vi "Teleop.vi"(10 "Match Info":T1={"Autonomous Elapsed Seconds"=0.0, "TeleOp Elapsed Seconds"=0.0, "Disabled Elapsed Seconds"=0.0, "Visited Autonomous"=FALSE, "Visited TeleOp"=FALSE, "Visited Disabled"=FALSE, "Autonomous Settings"={"Autonomous Style"=enum."Independent", "VI Refnum"=refnum}}, 11 "Call Context":T2) -> ()   [LabVIEW 2016]
doc: "This VI is called for each TeleOp packet received from the DS where the robot is not disabled. It is often used to read from the joysticks and update I/O or to update setpoints for timed control loops. It should complete and return within 20 milliseconds or it may miss DS packets."
uses:
  <vilib>/Rock Robotics/WPI/DriverStation/WPI_DriverStationDerivedRobotMode.ctl
  <vilib>/Rock Robotics/WPI/DriverStation/WPI_DriverStationMatch Info.ctl
  <vilib>/Rock Robotics/WPI/Solenoid/WPI_SolenoidValue.ctl
  <vilib>/Rock Robotics/WPI/Utilities/WPI_GetSetVariantRefNum.vi
  <vilib>/Rock Robotics/Network Tables/NT Read Boolean.vi
  <vilib>/Rock Robotics/WPI/Joystick/WPI_JoystickArcadeMapping.vi
  <vilib>/Rock Robotics/Network Tables/NT Write Number.vi
panel:
  out "Brake is Enabled 6":bool
  out "Brake is Enabled 5":bool
  out "Brake is Enabled 4":bool
  out "Brake is Enabled 3":bool
  out "Brake is Enabled 2":bool
  out "Brake is Enabled":bool
  out "Shift Status":dbl
  # "DRIVER CONTROLS"
  # "This is the number that is multiplied with the joystick output to determine high \ngear turning speed, the lower the number the slower it will turn in high gear."
  # "These numbers controls overall how sensitive the joystick is to turning and foreward\nmovement, the lower the number is the faster it will respond to joystick motion. \nIf the number is 1 then it will move in a linear relationship with the joystick."
  # "This controls the maximum foreward and backwards speed of the robot, if at 1 then\nthe robot can move at max power, if at 0 then the robot cannot move at all."
  # "This turns the ability to use autoshift on/off, if activated it does NOT mean that \nautoshift is always on, it simply means that it can be turned on with buttons 6/11."
  # "This turns the ability to use high gear on/off, if activated it does NOT mean that \nhigh gear is always on, it simply means that it can be turned on with button 1."
  # "This turns on the ability to reverse the direction of the robot with the buttons 8/9."
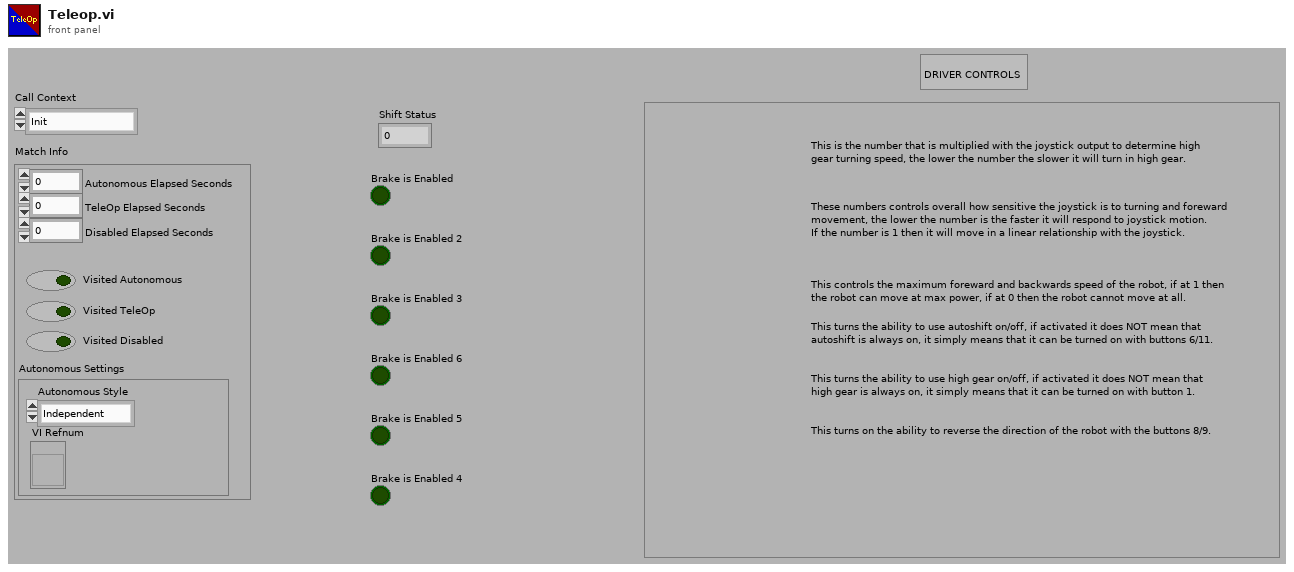
[diagram p1: front panel]
types:
  T1 = typedef "WPI_DriverStationMatch Info.ctl" = cluster{"Autonomous Elapsed Seconds":dbl, "TeleOp Elapsed Seconds":dbl, "Disabled Elapsed Seconds":dbl, "Visited Autonomous":bool, "Visited TeleOp":bool, "Visited Disabled":bool, "Autonomous Settings":cluster{"Autonomous Style":enum16{"Iterative", "Independent"}, "VI Refnum":refnum<vi>}}
  T2 = typedef "WPI_DriverStationDerivedRobotMode.ctl" = enum16{"Init", "Execute", "Stop"}
  T3 = typedef "WPI_JoystickDevRef.ctl" = cluster{"Device":T4}
  T4 = typedef "WPI_JoystickDeviceEnum.ctl" = enum16{"USB 0", "USB 1", "USB 2", "USB 3", "USB 4", "USB 5"}
  T5 = typedef "WPI_MotorControlDeviceRef.ctl" = cluster{"DeviceStatus":errorcluster, "Type":T6, "PWM":cluster{"PWM Channel":T7, "DeadBand":T8}, "CAN":cluster{"Device Number":u8, "SetOutput VI Ref":variant, "GetOutput VI Ref":variant, "Enable VI Ref":variant, "Disable VI Ref":variant, "Data":variant}, "Invert":bool}
  T6 = typedef "WPI_MotorControlType.ctl" = enum16{"PWM", "CAN"}
  T7 = typedef "FPGA_DIOPWMChannel.ctl" = enum8{"PWM 0", "PWM 1", "PWM 2", "PWM 3", "PWM 4", "PWM 5", "PWM 6", "PWM 7", "PWM 8", "PWM 9", "PWM MXP 0", "PWM MXP 1", "PWM MXP 2", "PWM MXP 3", "PWM MXP 4", "PWM MXP 5", "PWM MXP 6", "PWM MXP 7", "PWM MXP 8", "PWM MXP 9", "Invalid"}
  T8 = typedef "WPI_PWMDeadband.ctl" = cluster{"Name":string, "maxPositivePwm":i32, "minPositivePwm":i32, "centerPwm":i32, "maxNegativePwm":i32, "minNegativePwm":i32, "angularRange":u16}
  T9 = typedef "WPI_SolenoidDevRef.ctl" = cluster{"DevStatus":errorcluster, "Pneumatics Control Module":u8, "Forward Solenoid Channel":T10, "Reverse Solenoid Channel":T10}
  T10 = typedef "WPI_SolenoidChannel.ctl" = enum8{"Solenoid 0", "Solenoid 1", "Solenoid 2", "Solenoid 3", "Solenoid 4", "Solenoid 5", "Solenoid 6", "Solenoid 7", "Invalid"}
  T11 = typedef "WPI_CANTalonSRX_GlobalStatus.ctl" = cluster{"Applied Throttle":dbl, "Module Enabled":bool, "CAN Error":errorcluster, "Closed Loop Error":dbl, "Forward Limit Switch Closed":bool, "Reverse Limit Switch Closed":bool, "Sensor Position":dbl, "Sensor Velocity":dbl, "Current":dbl, "Sticky Fault - Over Temp":bool, "Sticky Fault - Under Voltage":bool, "Sticky Fault - Forward Limit":bool, "Sticky Fault - Reverse Limit":bool, "Sticky Fault - Forward Soft Limit":bool, "Sticky Fault - Reverse Soft Limit":bool, "Brake is Enabled":bool, "Encoder Position":dbl, "Encoder Velocity":dbl, "Encoder Index Count":dbl, "Encoder A Pin State":bool, "Encoder B Pin State":bool, "Encoder Index Pin State":bool, "Analog In":dbl, "Analog In Velocity":dbl, "Temperature (C)":dbl, "Battery Voltage":dbl, "Control 5 Is Supported":bool, "Current Profile Slot Select":dbl, "Pos Div 8":bool, "Vel Div 4":bool, "Pulse Width Position":i32, "Pulse Width Velocity":i32, "Pulse Width Rise To Rise (us)":i32, "Pulse Width Rise To Fall (us)":i32, "Mot Prof Active Is Under Run":bool, "Mot Prof Active Has Under Run":bool, "Mot Prof Active Is Last":bool, "Mot Prof Active Velocity Only":bool, "Mot Prof Active Is Valid":bool, "Mot Prof Buffer Is Full":bool, "Mot Prof Active Profile Slot Select":i32, "Mot Prof NextID":i32, "Mot Prof Count":i32, "Mot Prof Active Velocity":dbl, "Mot Prof Active Position":dbl, "Mot Prof Output Enable":i32}
  T12 = typedef "WPI_SolenoidValue.ctl" = enum16{"Off", "On", "Forward", "Reverse"}
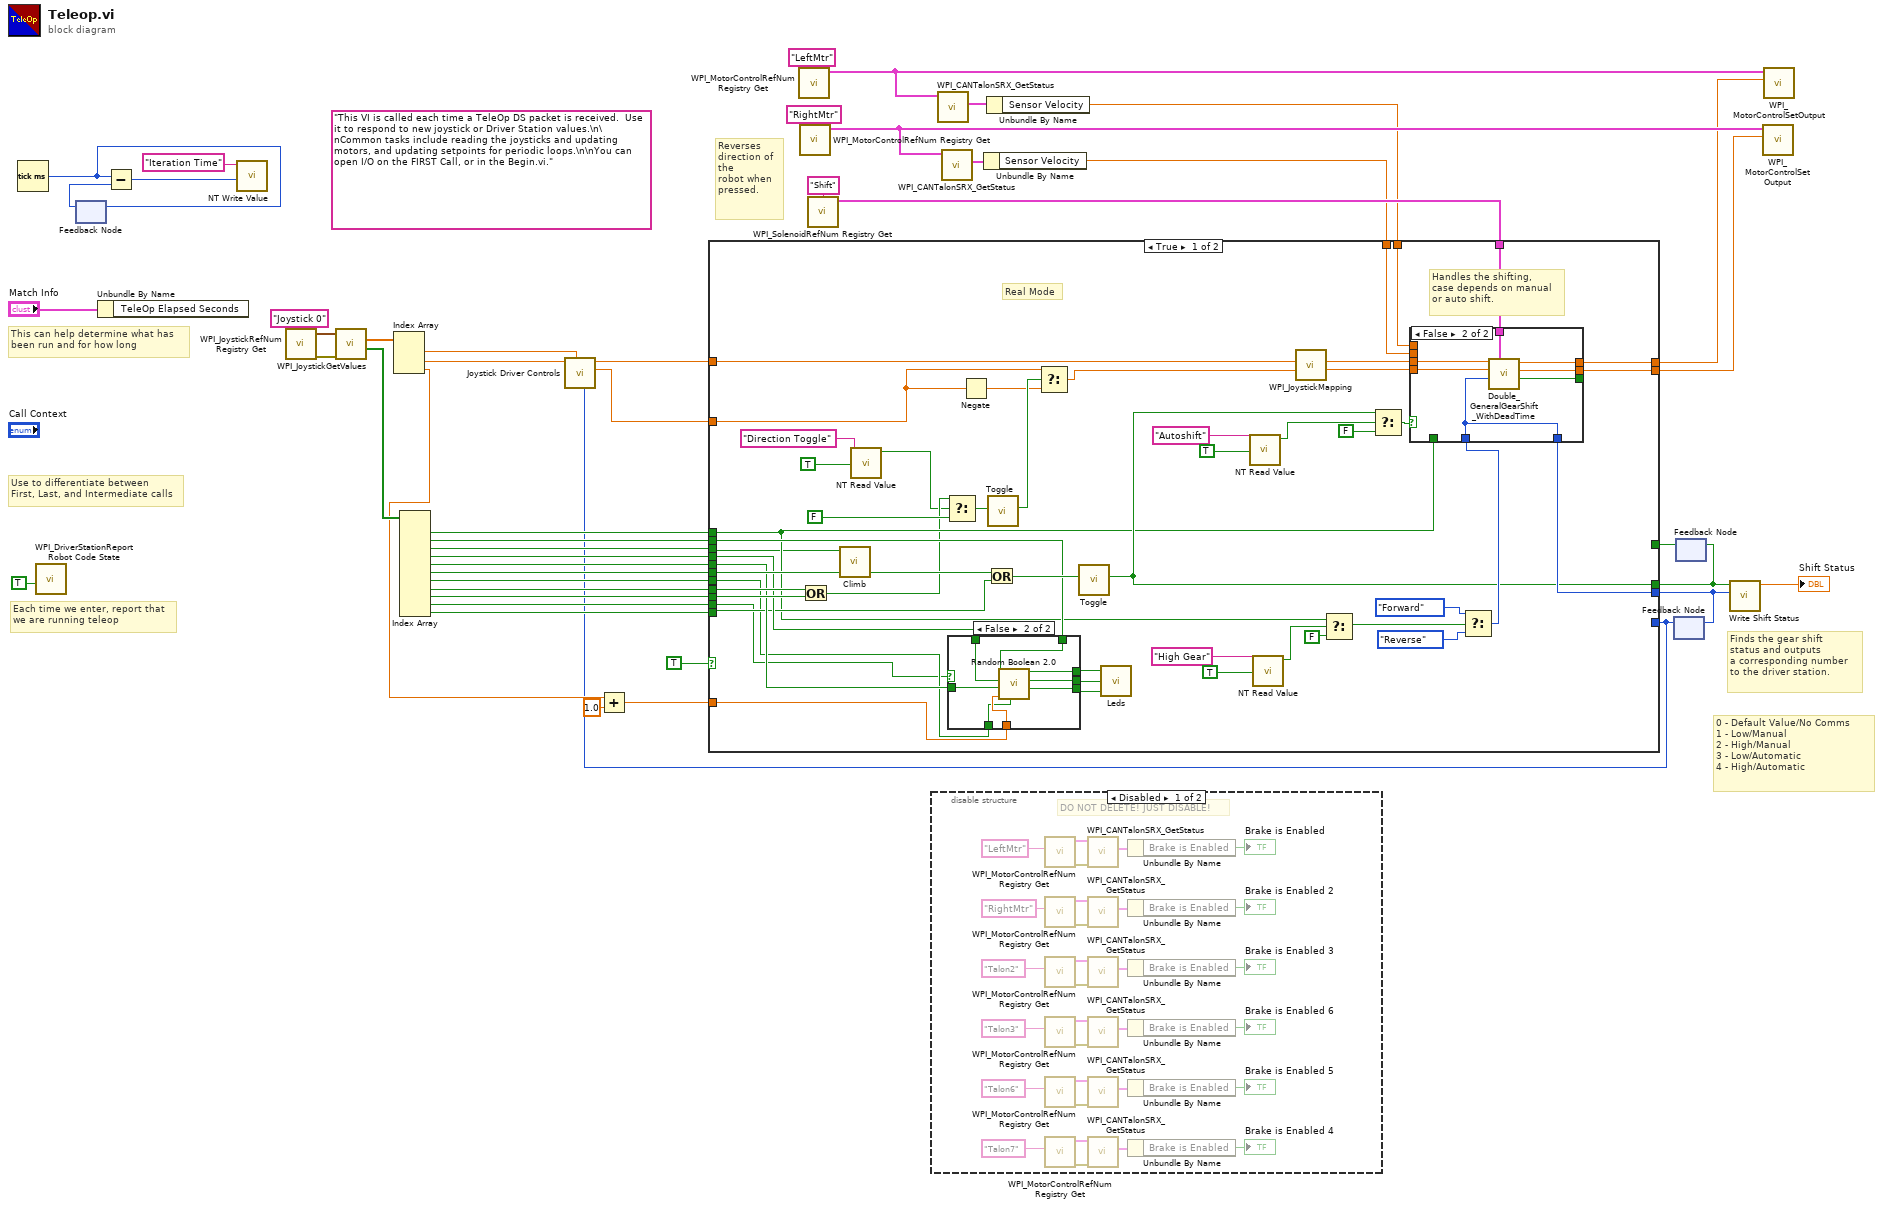
[diagram p0: block diagram]
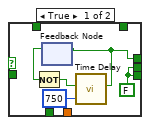
[diagram p2: hidden frame]
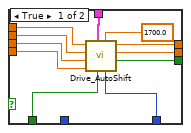
[diagram p3: hidden frame]
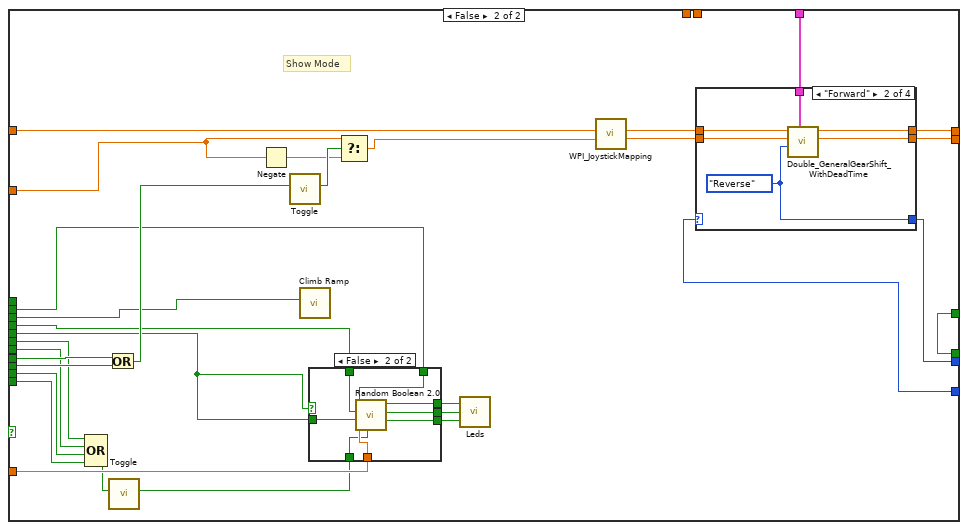
[diagram p4: hidden frame]
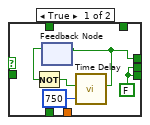
[diagram p5: hidden frame]
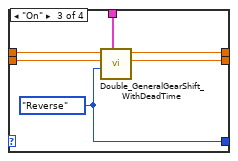
[diagram p7: hidden frame]
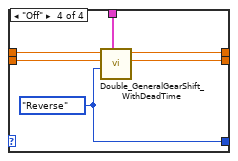
[diagram p8: hidden frame]
diagram:
  (unwired) "This VI is called each time a TeleOp DS packet is received.  Use it to respond to new joystick or Driver Station values.\n\nCommon tasks include reading the joysticks and updating motors, and updating setpoints for periodic loops.\n\nYou can open I/O on the FIRST Call, or in the Begin.vi."
  # "Reverses direction of the\nrobot when pressed."
  # "Finds the gear shift\nstatus and outputs\na corresponding number\nto the driver station."
  # "0 - Default Value/No Comms\n1 - Low/Manual\n2 - High/Manual\n3 - Low/Automatic\n4 - High/Automatic"
  # "Each time we enter, report that\nwe are running teleop"
  # "Use to differentiate between\nFirst, Last, and Intermediate calls"
  # "This can help determine what has\nbeen run and for how long"
  n1 = Tick Count (ms)() -> (millisecond timer value=w26:u32)
  n2 = call <vilib>:"WPI_DriverStationReport Robot Code State.vi"("TeleOp"=TRUE ("Autonomous")) -> ()  [unwired: 10 in, 1 out]
  n3 = feedback #1() -> (w27:u32)  [unwired: 1 in]
  n4 = feedback-in #1(w26) -> ()
  n5 = Unbundle By Name("Match Info") -> ()  [unwired: 1 out]
  n6 = Subtract(x=w26, y=w27) -> (x-y=w25:u32)
  n7 = call-poly <vilib>:"NT Write Value.vi"("Numeric"=w25, "Name"="Iteration Time") -> ()  [unwired: 9 in, 1 out]
  n8 = call <vilib>:"WPI_JoystickRefNum Registry Get.vi"("refnum name"="Joystick 0") -> ("error out"=w41:errorcluster, "JoystickDevRef"=w45:T3)  [unwired: 1 in, 8 out]
  n9 = call <vilib>:"WPI_JoystickGetValues.vi"("error in (no error)"=w41, "JoystickDevRef"=w45) -> ("Buttons"=w42:bool[], "Axes"=w43:dbl[])  [unwired: 5 in, 3 out]
  n10 = Index Array(array=w43) -> (element #1=w4:dbl, element #2=w3:dbl, element #3=w9:dbl)  [unwired: 3 in]
  n11 = Index Array(array=w42) -> (element #1=w16:bool, element #2=w12:bool, element #3=w17:bool, element #4=w11:bool, element #5=w10:bool, element #6=w36:bool, element #7=w37:bool, element #8=w39:bool, element #9=w40:bool, element #10=w19:bool, element #11=w18:bool)  [unwired: 11 in]
  n12 = Add(x=w9, y=1.0) -> (x+y=w8:dbl)
  n13 = call <vilib>:"WPI_MotorControlRefNum Registry Get.vi"("refnum name"="LeftMtr") -> ("MotorControlDevRef"=w34:T5)  [unwired: 9 in, 1 out]
  n14 = call <vilib>:"WPI_MotorControlRefNum Registry Get.vi"("refnum name"="RightMtr") -> ("MotorControlDevRef"=w33:T5)  [unwired: 9 in, 1 out]
  n15 = call <vilib>:"WPI_SolenoidRefNum Registry Get.vi"("refnum name"="Shift") -> ("SolenoidDevRef"=w35:T9)  [unwired: 9 in, 1 out]
  n16 = disable-structure shown="Disabled" {
    frame Disabled {
      # "DO NOT DELETE! JUST DISABLE!"
      n17 = call <vilib>:"WPI_MotorControlRefNum Registry Get.vi"("refnum name"="LeftMtr") -> ("error out"=w69:errorcluster, "MotorControlDevRef"=w70:T5)  [unwired: 9 in]
      n18 = call <vilib>:"WPI_MotorControlRefNum Registry Get.vi"("refnum name"="RightMtr") -> ("error out"=w55:errorcluster, "MotorControlDevRef"=w54:T5)  [unwired: 9 in]
      n19 = call <vilib>:"WPI_MotorControlRefNum Registry Get.vi"("refnum name"="Talon2") -> ("error out"=w57:errorcluster, "MotorControlDevRef"=w56:T5)  [unwired: 9 in]
      n20 = call <vilib>:"WPI_MotorControlRefNum Registry Get.vi"("refnum name"="Talon3") -> ("error out"=w53:errorcluster, "MotorControlDevRef"=w52:T5)  [unwired: 9 in]
      n21 = call <vilib>:"WPI_MotorControlRefNum Registry Get.vi"("refnum name"="Talon6") -> ("error out"=w50:errorcluster, "MotorControlDevRef"=w51:T5)  [unwired: 9 in]
      n22 = call <vilib>:"WPI_MotorControlRefNum Registry Get.vi"("refnum name"="Talon7") -> ("error out"=w48:errorcluster, "MotorControlDevRef"=w49:T5)  [unwired: 9 in]
      n23 = call <vilib>:"WPI_CANTalonSRX_GetStatus.vi"("error in (no error)"=w69, "CAN Talon SRX Ref"=w70) -> ("Talon SRX Status"=w71:T11)  [unwired: 7 in, 2 out]
      n24 = call <vilib>:"WPI_CANTalonSRX_GetStatus.vi"("error in (no error)"=w55, "CAN Talon SRX Ref"=w54) -> ("Talon SRX Status"=w66:T11)  [unwired: 7 in, 2 out]
      n25 = call <vilib>:"WPI_CANTalonSRX_GetStatus.vi"("error in (no error)"=w57, "CAN Talon SRX Ref"=w56) -> ("Talon SRX Status"=w65:T11)  [unwired: 7 in, 2 out]
      n26 = call <vilib>:"WPI_CANTalonSRX_GetStatus.vi"("error in (no error)"=w53, "CAN Talon SRX Ref"=w52) -> ("Talon SRX Status"=w58:T11)  [unwired: 7 in, 2 out]
      n27 = call <vilib>:"WPI_CANTalonSRX_GetStatus.vi"("error in (no error)"=w50, "CAN Talon SRX Ref"=w51) -> ("Talon SRX Status"=w61:T11)  [unwired: 7 in, 2 out]
      n28 = call <vilib>:"WPI_CANTalonSRX_GetStatus.vi"("error in (no error)"=w48, "CAN Talon SRX Ref"=w49) -> ("Talon SRX Status"=w62:T11)  [unwired: 7 in, 2 out]
      n29 = Unbundle By Name(w71) -> ("Brake is Enabled"=→"Brake is Enabled":bool)
      n30 = Unbundle By Name(w66) -> ("Brake is Enabled"=→"Brake is Enabled 2":bool)
      n31 = Unbundle By Name(w65) -> ("Brake is Enabled"=→"Brake is Enabled 3":bool)
      n32 = Unbundle By Name(w58) -> ("Brake is Enabled"=→"Brake is Enabled 6":bool)
      n33 = Unbundle By Name(w61) -> ("Brake is Enabled"=→"Brake is Enabled 5":bool)
      n34 = Unbundle By Name(w62) -> ("Brake is Enabled"=→"Brake is Enabled 4":bool)
    }
    frame Enabled {
    }
  }
  n35 = call <vilib>:"WPI_CANTalonSRX_GetStatus.vi"("CAN Talon SRX Ref"=w34) -> ("Talon SRX Status"=w21:T11)  [unwired: 8 in, 2 out]
  n36 = call <vilib>:"WPI_CANTalonSRX_GetStatus.vi"("CAN Talon SRX Ref"=w33) -> ("Talon SRX Status"=w20:T11)  [unwired: 8 in, 2 out]
  n37 = Unbundle By Name(w20) -> ("Sensor Velocity"=w32:dbl)
  n38 = Unbundle By Name(w21) -> ("Sensor Velocity"=w28:dbl)
  n39 = feedback #2() -> (w6:T12)  [unwired: 1 in]
  n40 = call "Joystick Driver Controls.vi"("Shift Value"=w6, "X"=w4, "Y"=w3) -> ("Y"=w2:dbl, "X"=w5:dbl)  [unwired: 7 in]
  n41 = feedback #3() -> (w13:bool)  [unwired: 1 in]
  n42 = case shown="True" TRUE {
    tunnel: w40 -> [w126 w176]
    tunnel: w39 -> [w125 w175]
    tunnel: w37 -> [w99 w166]
    tunnel: w36 -> [w118 w167]
    tunnel: w35 -> [w117 w180]
    tunnel: w32 -> [w116 _]
    tunnel: [w115 w181] -> w31
    tunnel: [w114 w183] -> w29
    tunnel: w28 -> [w113 _]
    tunnel: [w112 w179] -> w15
    tunnel: w19 -> [w98 w165]
    tunnel: w18 -> [w100 w164]
    tunnel: w17 -> [w78 w158]
    tunnel: w16 -> [w91 _]
    tunnel: [w95 w178] -> w14
    tunnel: w5 -> [w109 w160]
    tunnel: w2 -> [w108 w159]
    tunnel: w6 -> [_ w177]
    tunnel: w13 -> [_ w178]
    tunnel: w12 -> [w103 w170]
    tunnel: w11 -> [w102 w172]
    tunnel: w10 -> [w101 w161]
    tunnel: w8 -> [w104 w168]
    frame True {
      # "Real Mode"
      # "Handles the shifting,\ncase depends on manual\nor auto shift."
      n43 = Or(x=w125, y=w126) -> (x .or. y?=w88:bool)
      n44 = call "Climb.vi"("Climb"=w78) -> ()  [unwired: 11 in]
      n45 = call-poly <vilib>:"NT Read Value.vi"("Default Value"=TRUE, "Name"="Direction Toggle") -> ("Boolean"=w79:bool)  [unwired: 8 in, 1 out]
      n46 = Select(t=w88, s=w79, f=FALSE) -> (s? t:f=w89:bool)
      n47 = case shown="False" w98 {
        tunnel: w101 -> [_ w138]
        tunnel: [w131 w133] -> w105
        tunnel: w102 -> [_ w137]
        tunnel: [w131 w134] -> w106
        tunnel: w103 -> [_ w136]
        tunnel: [w130 w135] -> w107
        tunnel: w104 -> [_ w139]
        tunnel: w99 -> [_ w132]
        frame True {
          w131 = FALSE
          n48 = feedback #4() -> (w129:bool)  [unwired: 1 in]
          n49 = Not(x=w129) -> (.not. x?=w128:bool)
          n50 = call "Time Delay.vi"("Time Delay"=u32 750, "Boolean in"=w128) -> ("Boolean out"=w130:bool)  [unwired: 9 in]
          n51 = feedback-in #4(w130) -> ()
        }
        frame False {
          n52 = call "Random Boolean 2.0.vi"("Output Random"=w132, "Cycle Time"=w139, "Boolean in 3"=w138, "Boolean in 2"=w137, "Boolean in 1"=w136) -> ("Boolean out 3"=w133:bool, "Boolean out 2"=w134:bool, "Boolean out 1"=w135:bool)  [unwired: 4 in]
        }
      }
      n53 = Negate(x=w108) -> (-x=w111:dbl)
      n54 = Or(x=w118, y=w100) -> (x .or. y?=w110:bool)
      n55 = call "Toggle.vi"("Input"=w89) -> ("Output"=w120:bool)  [unwired: 10 in]
      n56 = Select(t=w108, s=w120, f=w111) -> (s? t:f=w119:dbl)
      n57 = call "Toggle.vi"("Input"=w110) -> ("Output"=w95:bool)  [unwired: 10 in]
      n58 = call "Leds.vi"("R"=w105, "G"=w106, "B"=w107) -> ()  [unwired: 1 in]
      n59 = call-poly <vilib>:"NT Read Value.vi"("Default Value"=TRUE, "Name"="Autoshift") -> ("Boolean"=w82:bool)  [unwired: 8 in, 1 out]
      n60 = call-poly <vilib>:"NT Read Value.vi"("Default Value"=TRUE, "Name"="High Gear") -> ("Boolean"=w85:bool)  [unwired: 8 in, 1 out]
      n61 = call-poly <vilib>:"WPI_JoystickMapping.vi"("Y axis value"=w119, "X axis value"=w109) -> ("Right Motor Value"=w121:dbl, "Left Motor Value"=w122:dbl)  [unwired: 8 in]
      n62 = Select(t=w91, s=w85, f=FALSE) -> (s? t:f=w92:bool)
      n63 = Select(t=w95, s=w82, f=FALSE) -> (s? t:f=w96:bool)
      n64 = Select(t=WPI_SolenoidValue."Forward" ("Value"), s=w92, f=WPI_SolenoidValue."Reverse" ("Value")) -> (s? t:f=w97:T12)
      n65 = case shown="False" w96 {
        tunnel: [w148 w157] -> w114
        tunnel: [w149 w156] -> w115
        tunnel: w122 -> [w147 w155]
        tunnel: w121 -> [w146 w154]
        tunnel: w117 -> [w142 w152]
        tunnel: [w150 w153] -> _
        tunnel: w116 -> [w145 _]
        tunnel: w113 -> [w144 _]
        tunnel: [w141 w151] -> w112
        tunnel: w97 -> [_ w151]
        tunnel: w91 -> [w140 _]
        frame True {
          n66 = call "Drive_AutoShift.vi"("Max"=1700.0, "Force Low Gear"=w140, "ShifterRef"=w142, "Right  Input"=w146, "Left Input"=w147, "Right RPM"=w145, "Left RPM"=w144) -> ("Shifting"=w150:bool, "Right Output"=w149:dbl, "Left Output"=w148:dbl, "Gear"=w141:T12)  [unwired: 1 in]
        }
        frame False {
          n67 = call "Double_GeneralGearShift_WithDeadTime.vi"("ShifterRef"=w152, "Shift Value"=w151, "Right"=w154, "Left"=w155) -> ("Shifting"=w153:bool, "Right Output"=w156:dbl, "Left Output"=w157:dbl)  [unwired: 4 in, 1 out]
        }
      }
    }
    frame False {
      # "Show Mode"
      n68 = Compound Arithmetic op=OR(w167, w166, w165, w164) -> (w163:bool)
      n69 = Or(x=w175, y=w176) -> (x .or. y?=w174:bool)
      n70 = call "Toggle.vi"("Input"=w163) -> ("Output"=w162:bool)  [unwired: 10 in]
      n71 = Negate(x=w159) -> (-x=w185:dbl)
      n72 = call "Toggle.vi"("Input"=w174) -> ("Output"=w187:bool)  [unwired: 10 in]
      n73 = call "Climb Ramp.vi"("Climb"=w158) -> ()  [unwired: 11 in]
      n74 = case shown="False" w161 {
        tunnel: w161 -> [_ w200]
        tunnel: [w192 w199] -> w173
        tunnel: w172 -> [_ w198]
        tunnel: [w192 w197] -> w171
        tunnel: w170 -> [_ w196]
        tunnel: [w191 w195] -> w169
        tunnel: w168 -> [_ w194]
        tunnel: w162 -> [_ w193]
        frame True {
          w192 = FALSE
          n75 = feedback #5() -> (w190:bool)  [unwired: 1 in]
          n76 = Not(x=w190) -> (.not. x?=w189:bool)
          n77 = call "Time Delay.vi"("Time Delay"=u32 750, "Boolean in"=w189) -> ("Boolean out"=w191:bool)  [unwired: 9 in]
          n78 = feedback-in #5(w191) -> ()
        }
        frame False {
          n79 = call "Random Boolean 2.0.vi"("Output Random"=w193, "Cycle Time"=w194, "Boolean in 3"=w200, "Boolean in 2"=w198, "Boolean in 1"=w196) -> ("Boolean out 3"=w199:bool, "Boolean out 2"=w197:bool, "Boolean out 1"=w195:bool)  [unwired: 4 in]
        }
      }
      n80 = Select(t=w159, s=w187, f=w185) -> (s? t:f=w186:dbl)
      n81 = call "Leds.vi"("R"=w173, "G"=w171, "B"=w169) -> ()  [unwired: 1 in]
      n82 = call-poly <vilib>:"WPI_JoystickMapping.vi"("Y axis value"=w186, "X axis value"=w160) -> ("Right Motor Value"=w182:dbl, "Left Motor Value"=w184:dbl)  [unwired: 8 in]
      n83 = case shown="\"Forward\"" w177 {
        selector: w177 -> [w201 _ _ _]
        tunnel: [w203 w206 w212 w218] -> w183
        tunnel: w184 -> [w203 w208 w214 w220]
        tunnel: w182 -> [w202 w207 w213 w219]
        tunnel: [w202 w205 w211 w217] -> w181
        tunnel: w180 -> [_ w209 w215 w221]
        tunnel: [w201 w204 w210 w216] -> w179
        frame "Reverse", Default {
        }
        frame "Forward" {
          w204 = WPI_SolenoidValue."Reverse" ("Shift Value")
          n84 = call "Double_GeneralGearShift_WithDeadTime.vi"("ShifterRef"=w209, "Shift Value"=w204, "Right"=w207, "Left"=w208) -> ("Right Output"=w205:dbl, "Left Output"=w206:dbl)  [unwired: 4 in, 2 out]
        }
        frame "On" {
          w210 = WPI_SolenoidValue."Reverse" ("Shift Value")
          n85 = call "Double_GeneralGearShift_WithDeadTime.vi"("ShifterRef"=w215, "Shift Value"=w210, "Right"=w213, "Left"=w214) -> ("Right Output"=w211:dbl, "Left Output"=w212:dbl)  [unwired: 4 in, 2 out]
        }
        frame "Off" {
          w216 = WPI_SolenoidValue."Reverse" ("Shift Value")
          n86 = call "Double_GeneralGearShift_WithDeadTime.vi"("ShifterRef"=w221, "Shift Value"=w216, "Right"=w219, "Left"=w220) -> ("Right Output"=w217:dbl, "Left Output"=w218:dbl)  [unwired: 4 in, 2 out]
        }
      }
    }
  }
  n87 = feedback-in #2(w15) -> ()
  n88 = feedback-in #3(w14) -> ()
  n89 = call "Write Shift Status.vi"("Gear"=w15, "Output"=w14) -> ("Shift Status"=→"Shift Status":dbl)  [unwired: 9 in]
  n90 = call <vilib>:"WPI_MotorControlSetOutput.vi"("Output"=w31, "MotorControlDevRef"=w33) -> ()  [unwired: 7 in, 3 out]
  n91 = call <vilib>:"WPI_MotorControlSetOutput.vi"("Output"=w29, "MotorControlDevRef"=w34) -> ()  [unwired: 7 in, 3 out]
